vi "Functional Imaging-Refresh UI.vi"(6 "Select the first element":bool, 7 "Reset graph X-axis scaling (F)":bool, 8 "error in (no error)":errorcluster) -> ()   [LabVIEW 2020]
uses:
  Typedefs/Overlay FG functions.ctl
  Global variables/gl_Functional Imaging-Global variables.vi
panel:
  out "X-axis max/min (across all loaded data types)":cluster{"X-axis max":dbl, "X-axis min":dbl}
  out "Total # of loaded points":i32
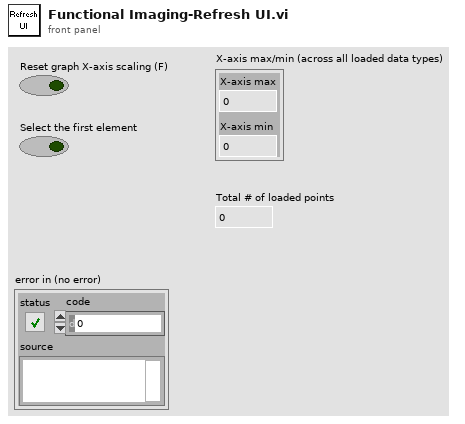
[diagram p1: front panel]
types:
  T1 = typedef "Overlay FG functions.ctl" = enum16{"Generate new images", "Get stored images", "Clear"}
  T2 = typedef "IMAQ Image.ctl" = refnum<image>
  T3 = typedef "Functional Imging UI Refs.ctl" = cluster{"Menu ref":refnum<k9>, "Image control":refnum<vi>, "VI ref":refnum<vi>, "XGrapher":refnum<vi>, "Smoothing":refnum<vi>, "POI Averaging":refnum<vi>, "Normalize":refnum<vi>, "POI data points in each trial":refnum<vi>, "Channel":refnum<vi>, "Experiment data folder path":refnum<vi>, "[ROI vis]":refnum<vi>, "[Groups] visbl":T4, "Group Name":refnum<vi>, "POI index":refnum<vi>, "Trial No.":refnum<vi>, "Intensity Zoom":refnum<vi>, "Trial Cursor Enabled":refnum<vi>, "Number of Trials (ind 1)":refnum<vi>, "Number of Trials (ind 2)":refnum<vi>, "MiniScans Available":refnum<vi>, "POI Available":refnum<vi>, "Defer graph updates":refnum<vi>, "Waveform selector":refnum<vi>, "#of selected POI":refnum<vi>, "#of selected MiniScans":refnum<vi>, "#of selected groups":refnum<vi>, "Max Z-Projection":refnum<vi>, "Z-Plane Selector":refnum<vi>, "Index of miniscan point to visualise":refnum<vi>, "ROI vis. mode":refnum<vi>, "Total # of points":refnum<vi>, "Index of group clicked on":refnum<vi>, "Pane 1":refnum<vi>, "Pane 2":refnum<vi>, "Pane 3":refnum<vi>, "Pane 4":refnum<vi>, "Pane 5":refnum<vi>, "Pane 6":refnum<vi>, "Deselect all ROI":refnum<vi>, "Deselect all groups":refnum<vi>}
  T4 = typedef "Groups array referecne.ctl" = refnum<vi>
  T5 = typedef "Interface-ROI type enum.ctl" = enum16{"POI", "Mini-scan"}
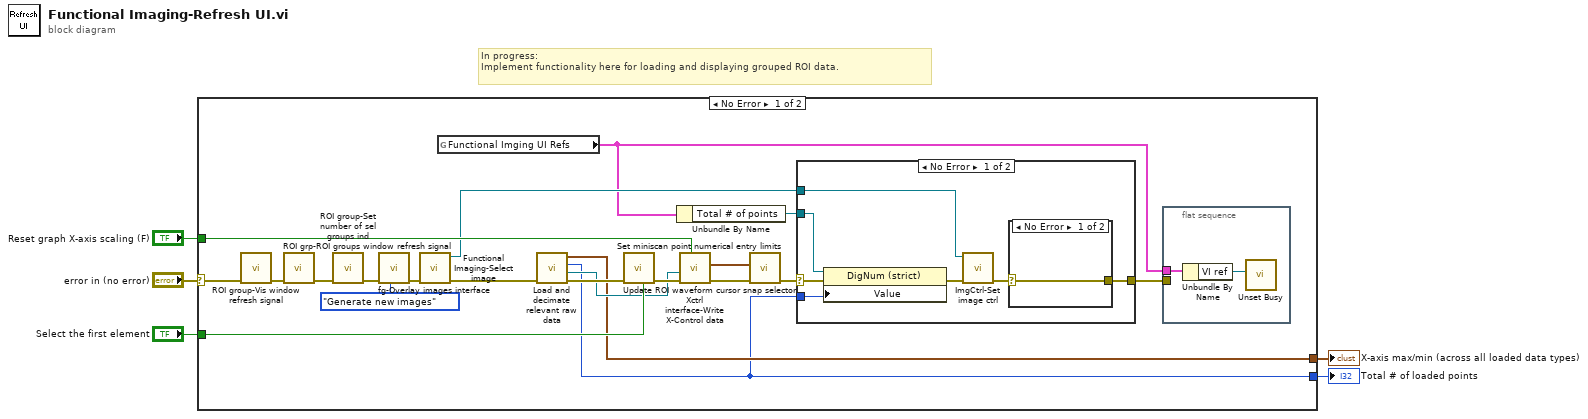
[diagram p0: block diagram]
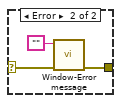
[diagram p2: hidden frame]
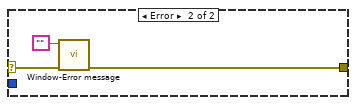
[diagram p3: hidden frame]
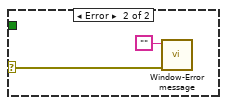
[diagram p4: hidden frame]
diagram:
  # "In progress:\nImplement functionality here for loading and displaying grouped ROI data."
  n1 = case shown="No Error" "error in (no error)" {
    selector: "error in (no error)" -> [w14 w43]
    tunnel: [w9 _] -> w5
    tunnel: [w10 _] -> w4
    tunnel: "Reset graph X-axis scaling (F)" -> [w24 _]
    tunnel: "Select the first element" -> [w22 _]
    frame No Error {
      n2 = call "ROI group-Vis window refresh signal.vi"("error in (no error)"=w14) -> ("error out"=w13:errorcluster)  [unwired: 10 in]
      n3 = call "ROI grp-ROI groups window refresh signal.vi"("error in (no error)"=w13) -> ("error out"=w15:errorcluster)  [unwired: 10 in]
      n4 = call "ROI group-Set number of sel groups ind.vi"("error in (no error)"=w15) -> ("error out"=w16:errorcluster)  [unwired: 10 in]
      n5 = call "fg-Overlay images interface.vi"("Function"=Overlay_FG_functions."Generate new images", "error in (no error)"=w16) -> ("error out"=w26:errorcluster)  [unwired: 7 in, 2 out]
      n6 = call "Functional Imaging-Select image.vi"("error in (no error)"=w26) -> ("error out"=w8:errorcluster, "SelectedPOIMax"=w18:T2)  [unwired: 9 in]
      n7 = global read "gl_Functional Imaging-Global variables.vi" "Functional Imging UI Refs"() -> (w7:T3)
      n8 = call "Load and decimate relevant raw data.vi"("error in (no error)"=w8) -> ("error out"=w12:errorcluster, "Data reference"=w11:refnum<data-value>, "Total # of loaded points"=w9:i32, "X-axis max/min (across all loaded data types)"=w10:cluster{"X-axis max":dbl, "X-axis min":dbl})  [unwired: 7 in]
      n9 = call "Update ROI waveform cursor snap selector.vi"("Reset selection to the first element"=w22, "error in (no error)"=w12) -> ("error out"=w23:errorcluster)  [unwired: 9 in]
      n10 = Unbundle By Name(w7) -> ("Total # of points"=w19:refnum<vi>)
      n11 = call "Xctrl interface-Write X-Control data.vi"("Reset graph X-axis scaling (F)"=w24, "error in (no error)"=w23, "Data reference"=w11) -> ("error out"=w21:errorcluster, "Properties of selected ROI"=w20:cluster{"Type":T5, "Points per cycle":u16})  [unwired: 7 in]
      n12 = call "Set miniscan point numerical entry limits.vi"("error in"=w21, "Properties of selected ROI"=w20) -> ("error out"=w17:errorcluster)  [unwired: 9 in]
      n13 = case shown="No Error" w17 {
        selector: w17 -> [w32 w41]
        tunnel: w18 -> [w34 _]
        tunnel: w9 -> [w35 _]
        tunnel: w19 -> [w33 _]
        tunnel: [w29 w40] -> w6
        frame No Error {
          n14 = property on="Property Node" class="DigNum (strict)"(reference=w33, error in=w32, "Value"=w35) -> (error out=w31:errorcluster)  [unwired: 1 out]
          n15 = call "ImgCtrl-Set image ctrl.vi"("error in"=w31, "Image"=w34) -> ("error out"=w30:errorcluster)  [unwired: 9 in]
          n16 = case shown="No Error" w30 {
            selector: w30 -> [w36 w38]
            tunnel: [w36 w37] -> w29
            frame No Error {
            }
            frame Error {
              n17 = call "Window-Error message.vi"("error in (no error)"=w38, "Message"="") -> ("Error Out (no error)"=w37:errorcluster)  [unwired: 9 in]
            }
          }
        }
        frame Error {
          n18 = call "Window-Error message.vi"("error in (no error)"=w41, "Message"="") -> ("Error Out (no error)"=w40:errorcluster)  [unwired: 9 in]
        }
      }
      n19 = flat-sequence {
        tunnel: w7 -> [w27]
        tunnel: w6 -> [_]
        frame #0 {
          n20 = Unbundle By Name(w27) -> ("VI ref"=w28:refnum<vi>)
          n21 = call <vilib>:"Unset Busy.vi"("VI reference (current VI)"=w28) -> ()  [unwired: 10 in, 1 out]
        }
      }
    }
    frame Error {
      n22 = call "Window-Error message.vi"("error in (no error)"=w43, "Message"="") -> ()  [unwired: 9 in, 1 out]
    }
  }
  "Total # of loaded points" <- w5
  "X-axis max/min (across all loaded data types)" <- w4
